vi "NewDialog.vi"(6 "inIcon":T1(ring), 7 "inTitle":string, 8 "inButton3Text":string="Cancel", 9 "inButton2Text":string="OK", 10 "inButton1Text":string="OK", 11 "inMessage":string="I can write these many sentences without any problem, else I could try this and that and without doubt only some of these characters would fit. It may happen that in case of any minor inconveniences, that a person may get somewhat discouraged, but this is as expected and often has no bearing on any final outcomes. As it turns out!") -> (1 "outButton3":bool, 2 "outButton2":bool, 3 "outButton1":bool)   [LabVIEW 2021]
doc: "v3:\n- VI opens only after data is loaded/updated \n\nTitle: Heading of Message\n\nIcon: Symbol for heading of message; see enum\n\nButton1: One-button dialog type; text on button. NOTE: This field should be left em[pty in case of two button dialog equirement\n\nButton2: Left button text in a two-button dialog type\n\nButton3: Right button text in a two-button dialog type"
panel:
  out "Tab Control":enum32{"Single", "Double"}(tab)
  in  "Button1":bool
  in  "Button2":bool caption="Button1"
  in  "Button3":bool caption="Button1"
  out "Title":string="GENERAL\nERROR" caption="Pump Feeder:Operation Timed Out: Wait For Parts 2"
  out "Ring":u8(ring)=7
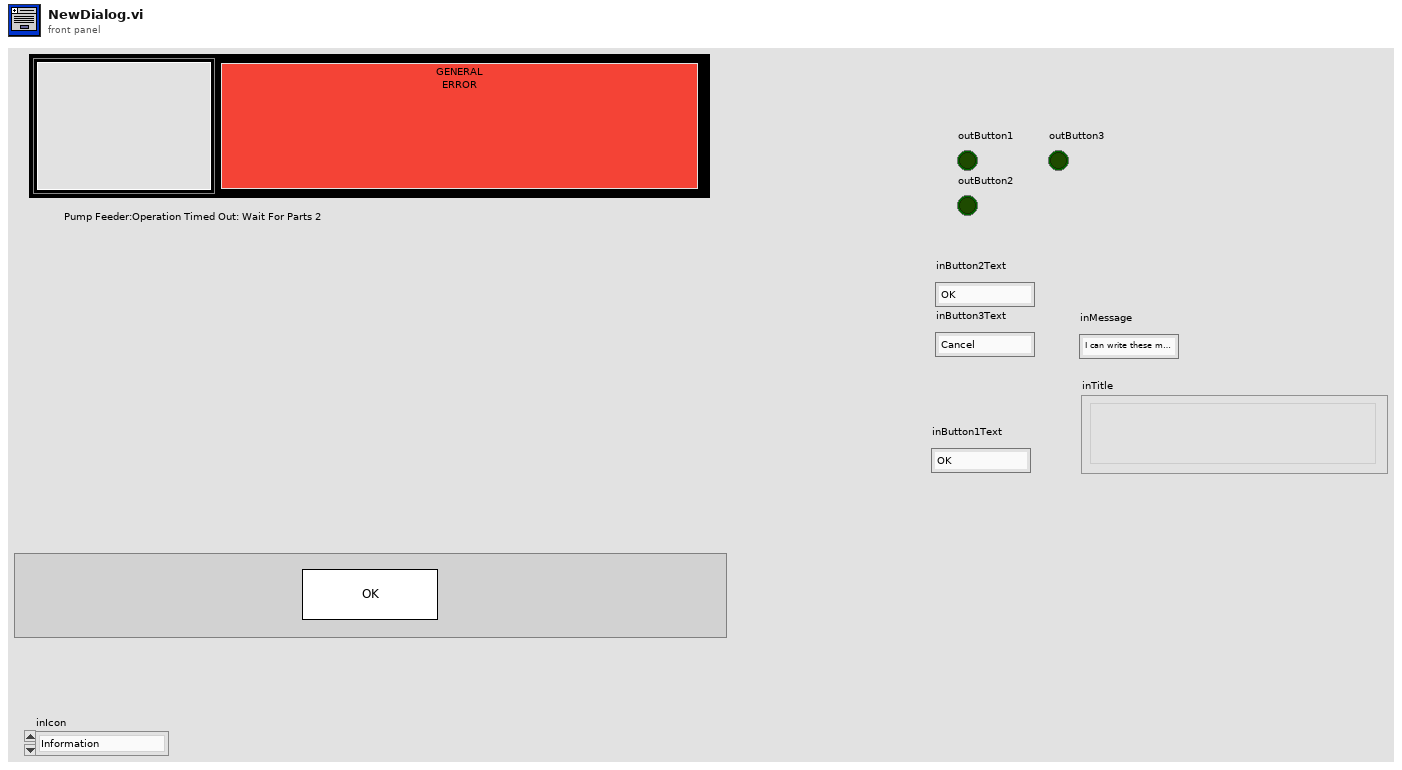
[diagram p1: front panel]
types:
  T1 = enum8{"Information", "Error", "Successful", "Tips"}
  T2 = enum32{"Invalid", "Standard", "Closed", "Hidden", "Minimized", "Maximized"}
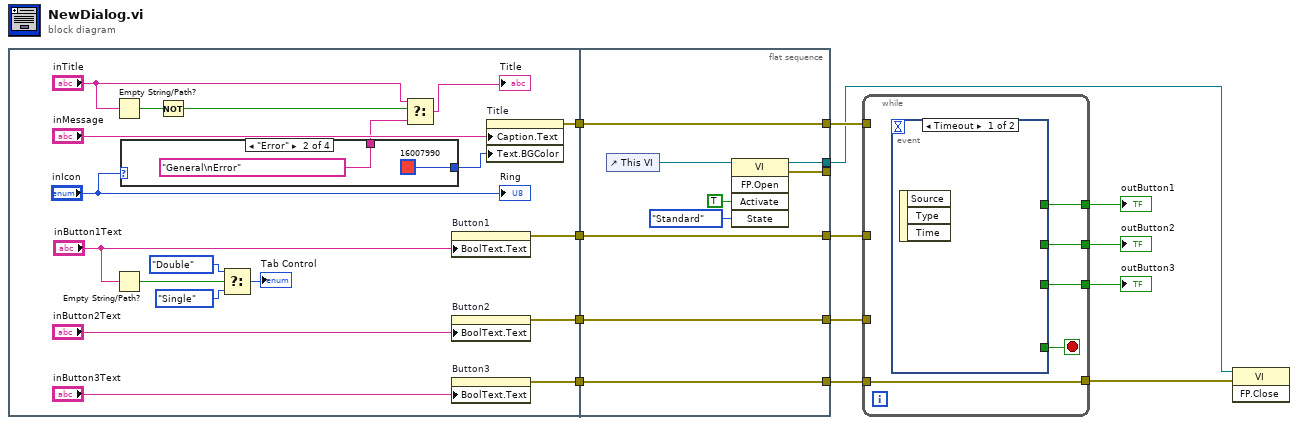
[diagram p0: block diagram]
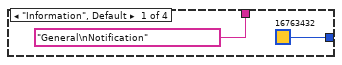
[diagram p2: hidden frame]
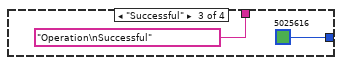
[diagram p3: hidden frame]
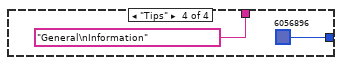
[diagram p4: hidden frame]
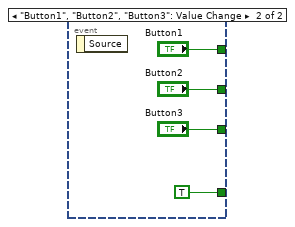
[diagram p5: hidden frame]
diagram:
  n1 = flat-sequence {
    tunnel: [w18] -> w6
    tunnel: [w17] -> w5
    tunnel: [w16] -> w4
    tunnel: [w15] -> w3
    tunnel: [w46] -> w7
    tunnel: [w47] -> w8
    tunnel: [w48] -> w9
    tunnel: [w49] -> w10
    tunnel: w6 -> [w49]
    tunnel: w5 -> [w48]
    tunnel: w4 -> [w47]
    tunnel: w3 -> [w46]
    tunnel: [w42] -> _
    tunnel: [w41] -> w2
    frame #0 {
      n2 = Empty String/Path?(string/path="inTitle") -> (empty?=w22:bool)
      n3 = Empty String/Path?(string/path="inButton1Text") -> (empty?=w24:bool)
      n4 = case shown="\"Error\"" "inIcon" {
        tunnel: [u32 16763432 u32 16007990 u32 5025616 u32 6056896] -> w20
        tunnel: ["General\nNotification" "General\nError" "Operation\nSuccessful" "General\nInformation"] -> w14
        frame "Information", Default {
        }
        frame "Error" {
        }
        frame "Successful" {
        }
        frame "Tips" {
        }
      }
      n5 = Not(x=w22) -> (.not. x?=w21:bool)
      n6 = Select(t=enum32{"Single", "Double"}."Double" ("Tab Control"), s=w24, f=enum32{"Single", "Double"}."Single" ("Tab Control")) -> (s? t:f=→"Tab Control":enum32{"Single", "Double"})
      n7 = Select(t="inTitle", s=w21, f=w14) -> (s? t:f=→"Title":string)
      n8 = property on="Button1" class="Bool"("BoolText.Text"="inButton1Text") -> (error out=w17:errorcluster)  [unwired: 2 in, 1 out]
      n9 = property on="Button2" class="Bool"("BoolText.Text"="inButton2Text") -> (error out=w16:errorcluster)  [unwired: 2 in, 1 out]
      n10 = property on="Button3" class="Bool"("BoolText.Text"="inButton3Text") -> (error out=w15:errorcluster)  [unwired: 2 in, 1 out]
      n11 = property on="Title" class="Str"("Caption.Text"="inMessage", "Text.BGColor"=w20) -> (error out=w18:errorcluster)  [unwired: 2 in, 1 out]
      "Ring" <- "inIcon"
    }
    frame #1 {
      n12 = control-ref of="This VI"() -> (w43:refnum<vi>)
      n13 = invoke class="VI" method="FP.Open"(reference=w43, "Activate"=TRUE ("Activate?"), "State"=T2."Standard") -> (reference out=w41:refnum<vi>, error out=w42:errorcluster)  [unwired: 2 in, 3 out]
    }
  }
  n14 = while {
    tunnel: [w54] -> w13
    tunnel: [w53] -> w12
    tunnel: [w52] -> w11
    tunnel: w10 -> [_]
    tunnel: w9 -> [_]
    tunnel: w8 -> [_]
    tunnel: w7 -> [w50]
    tunnel: [w50] -> w1
    stop <- w51 stop-if-true
    n15 = event shown="[0] Timeout" {
      selector: _ -> [_ _]
      dyn-events: _ -> [_ _]
      timeout: _ -> [_ _]
      tunnel: [_ "Button1"] -> w54
      tunnel: [_ "Button2"] -> w53
      tunnel: [_ "Button3"] -> w52
      tunnel: [_ TRUE] -> w51
      event Timeout {
        n16 = event-data() -> ()  [unwired: 1 in, 3 out]
      }
      event "Button1", "Button2", "Button3": Value Change {
        n17 = event-data() -> ()  [unwired: 1 in, 1 out]
      }
    }
  }
  "outButton1" <- w13
  "outButton2" <- w12
  "outButton3" <- w11
  n18 = invoke class="VI" method="FP.Close"(reference=w2, error in=w1) -> ()  [unwired: 1 in, 3 out]
